vi "Model - Get Account Number.vi"(8 "error in (no error)":errorcluster, 11 "View Model":T1) -> (0 "error out":errorcluster, 2 "Account Number":u32, 3 "View Model":T1)   [LabVIEW 2017]
doc: "Get actual values of Account Number from DVR."
uses:
  Controls/View Model.ctl
  Controls/Shared Model.ctl
  Error Handler/Controls/Error Model.ctl
  Error Handler/Controls/Error Data.ctl
  Error Handler/Controls/Error Type.ctl
  Error Handler/Controls/Error Source.ctl
  Configuration/Controls/Config Model.ctl
  Configuration/Controls/Config CMD.ctl
  Configuration/Controls/Config Command.ctl
  Controller/Controls/Controller Model.ctl
  Controller/Controls/Controller Overhead.ctl
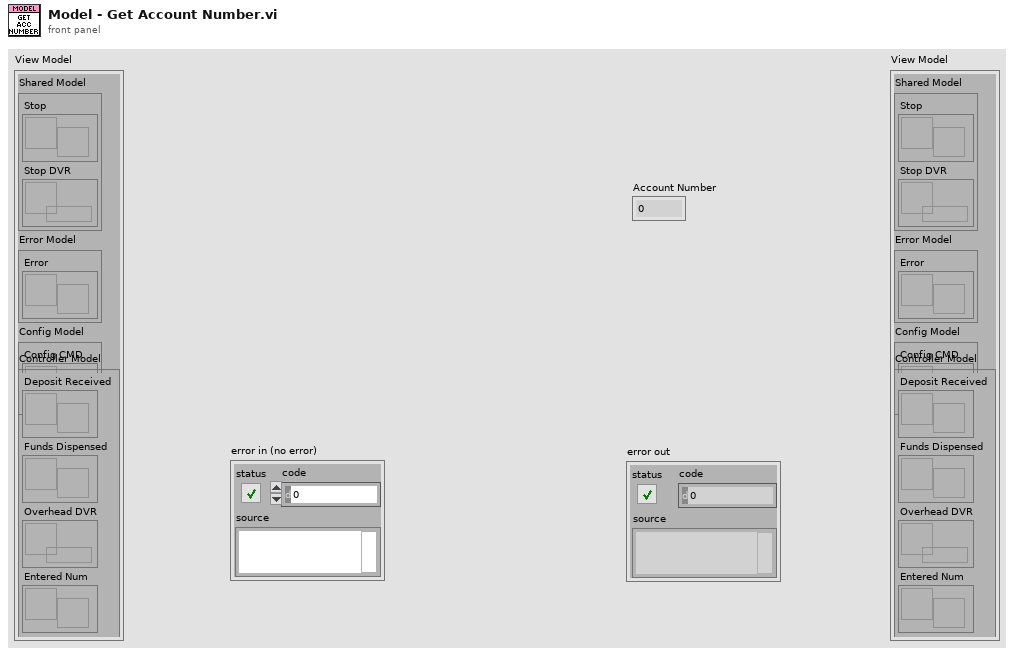
[diagram p1: front panel]
types:
  T1 = typedef "View Model.ctl" = cluster{"Shared Model":T2, "Error Model":T3, "Config Model":T4, "Controller Model":T5}
  T2 = typedef "Shared Model.ctl" = cluster{"Stop":refnum<user-event>, "Stop DVR":refnum<data-value>}
  T3 = typedef "Error Model.ctl" = cluster{"Error":refnum<user-event>}
  T4 = typedef "Config Model.ctl" = cluster{"Config CMD":refnum<user-event>}
  T5 = typedef "Controller Model.ctl" = cluster{"Deposit Received":refnum<user-event>, "Funds Dispensed":refnum<user-event>, "Overhead DVR":refnum<data-value>, "Entered Num":refnum<user-event>, "Card Read":refnum<user-event>}
  T6 = typedef "Controller Overhead.ctl" = cluster{"Current Transaction":string, "Message":string, "Card Read":bool, "Account Number":u32, "Amount":u32}
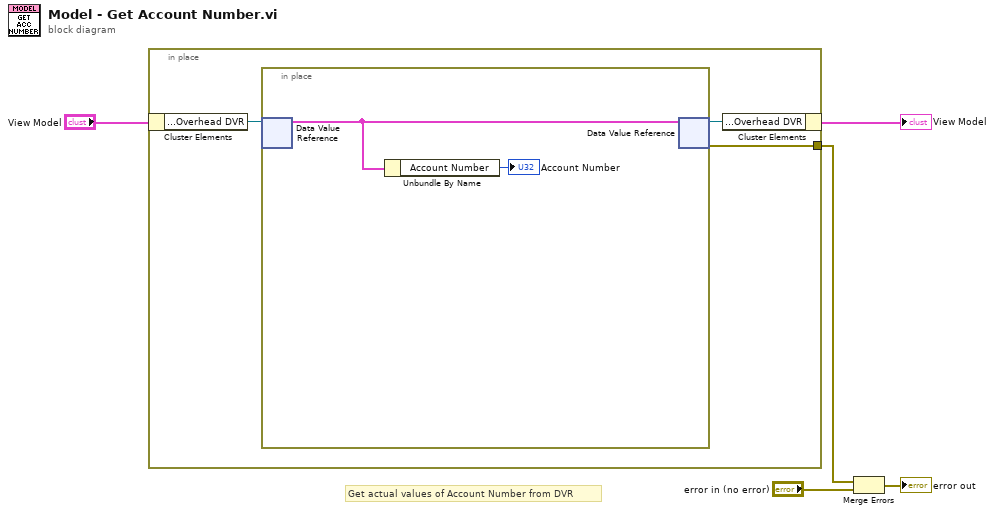
[diagram p0: block diagram]
diagram:
  # "Get actual values of Account Number from DVR"
  n1 = in-place {
    in-place-border: [w6] -> w3
    n2 = in-place-cluster #1("View Model") -> ("Controller Model.Overhead DVR"=w8:refnum<data-value>)
    n3 = in-place {
      n4 = in-place-dvr #2(w8) -> (w10:T6)  [unwired: 1 out]
      n5 = Unbundle By Name(w10) -> ("Account Number"=→"Account Number":u32)
      n6 = in-place-dvr #2(w10) -> (w7:refnum<data-value>, w6:errorcluster)
    }
    n7 = in-place-cluster #1("Controller Model.Overhead DVR"=w7) -> (→"View Model":T1)
  }
  n8 = Merge Errors(w3, "error in (no error)") -> (→"error out":errorcluster)
